vi "点至线段的角平分线点.vi"(8 "Error In":errorcluster caption="错误输入", 10 "线段":T2, 11 "点A":T1 caption="点（双精度）") -> (0 "Error Out":errorcluster caption="错误输出", 3 "角平分线点":T1)   [LabVIEW 2015, in "几何工具.lvlib"]
uses:
  <vilib>/Utility/miscctls.llb/LVPointDoubleTypeDef.ctl
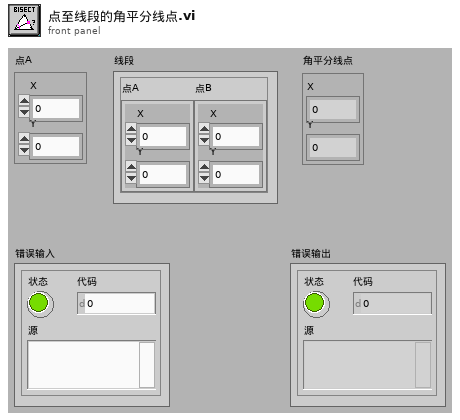
[diagram p1: front panel]
types:
  T1 = typedef "LVPointDoubleTypeDef.ctl" = cluster{"X":dbl, "Y":dbl}
  T2 = typedef "两点直线.ctl" = cluster{"点A":T1, "点B":T1}
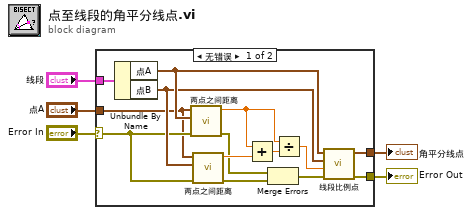
[diagram p0: block diagram]
diagram:
  n1 = case shown="无错误" "Error In" {
    selector: "Error In" -> [w12 w20]
    tunnel: [w13 _] -> w4
    tunnel: [w10 w20] -> w3
    tunnel: "线段" -> [w9 _]
    tunnel: "点A" -> [w8 _]
    frame No Error {
      n2 = Unbundle By Name(w9) -> ("点A"=w16:T1, "点B"=w15:T1)
      n3 = call "两点之间距离.vi"("Error In"=w12, "点B"=w16, "点A"=w8) -> ("Error Out"=w6:errorcluster, "距离AB"=w17:dbl)  [unwired: 7 in]
      n4 = call "两点之间距离.vi"("Error In"=w12, "点B"=w15, "点A"=w8) -> ("Error Out"=w11:errorcluster, "距离AB"=w19:dbl)  [unwired: 7 in]
      n5 = Add(x=w17, y=w19) -> (x+y=w18:dbl)
      n6 = Merge Errors(w6, w11) -> (w7:errorcluster)
      n7 = Divide(x=w17, y=w18) -> (x/y=w14:dbl)
      n8 = call "线段比例点.vi"("Error In"=w7, "比例(CA/AB)"=w14, "点B"=w15, "点A"=w16) -> ("Error Out"=w10:errorcluster, "比例点"=w13:T1)  [unwired: 6 in]
    }
    frame Error {
    }
  }
  "Error Out" <- w3
  "角平分线点" <- w4
